vi "Rewind.vi"(10 "State (No Change)":T1, 11 "Constructor String Parser In":T2) -> (3 "Constructor String Parser":T2)   [LabVIEW 2020, in "Stream.lvlib" / "URLPattern.lvclass"]
uses:
  URLPattern.lvclass
  Constructor String Parser.ctl
  Token.ctl
  Token Type.ctl
  URL Pattern Init.ctl
  Parser State.ctl
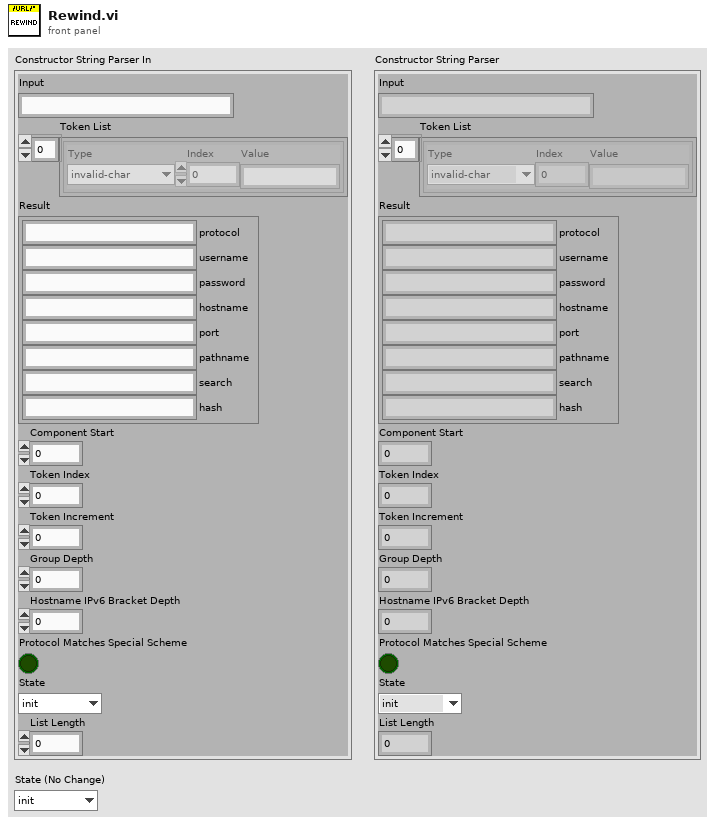
[diagram p1: front panel]
types:
  T1 = typedef "Stream.lvlib/URLPattern.lvclass/Parser State.ctl" = enum16{"init", "protocol", "authority", "username", "password", "hostname", "port", "pathname", "search", "hash", "done"}
  T2 = typedef "Stream.lvlib/URLPattern.lvclass/Constructor String Parser.ctl" = cluster{"Input":string, "Token List":T3[], "Result":T5, "Component Start":i32, "Token Index":i32, "Token Increment":i32, "Group Depth":i32, "Hostname IPv6 Bracket Depth":i32, "Protocol Matches Special Scheme":bool, "State":T1, "List Length":i32}
  T3 = typedef "Stream.lvlib/URLPattern.lvclass/Token.ctl" = cluster{"Type":T4, "Index":i32, "Value":string}
  T4 = typedef "Stream.lvlib/URLPattern.lvclass/Token Type.ctl" = enum16{"invalid-char", "open", "close", "regexp", "name", "char", "escaped-char", "other-modifier", "asterisk", "end"}
  T5 = typedef "Stream.lvlib/URLPattern.lvclass/URL Pattern Init.ctl" = cluster{"protocol":string, "username":string, "password":string, "hostname":string, "port":string, "pathname":string, "search":string, "hash":string}
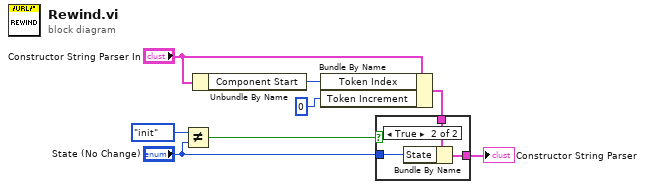
[diagram p0: block diagram]
diagram:
  n1 = Not Equal?(x=Parser_State."init" ("y"), y="State (No Change)") -> (x != y?=w4:bool)
  n2 = Unbundle By Name("Constructor String Parser In") -> ("Component Start"=w7:i32)
  n3 = Bundle By Name(cluster="Constructor String Parser In", "Token Index"=w7, "Token Increment"=0) -> (w2:T2)
  n4 = case shown="True" w4 {
    tunnel: "State (No Change)" -> [_ w12]
    tunnel: w2 -> [w9 w11]
    tunnel: [w9 w10] -> w1
    frame False {
    }
    frame True {
      n5 = Bundle By Name(cluster=w11, "State"=w12) -> (w10:T2)
    }
  }
  "Constructor String Parser" <- w1
